vi "Date Stamp.vi"(1 "Format (12 Digit ymdHMS)":string="%Y-%m-%d %H_%M_%S") -> (4 "String Out":string, 5 "U64 Out":u64)   [LabVIEW 2015]
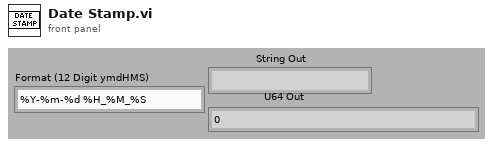
[diagram p1: front panel]
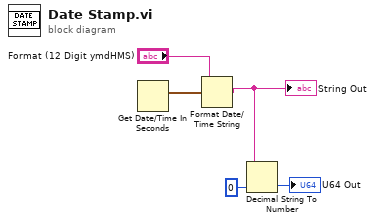
[diagram p0: block diagram]
diagram:
  n1 = Get Date/Time In Seconds() -> (seconds since 1Jan1904=w4:timestamp)
  n2 = Format Date/Time String(time format string (%c)="Format (12 Digit ymdHMS)", seconds (now)=w4) -> (date/time string=w1:string)  [unwired: 1 in]
  "String Out" <- w1
  n3 = Decimal String To Number(string=w1, default (0L)=u64 0 ("default (0 I32)")) -> (number=→"U64 Out":u64)  [unwired: 1 in, 1 out]
